vi "plot_digital.vi"(9 "array":dbl[](array[numeric]), 10 "Outputs":T1(array[cluster])=[{"Output"=0, "Offset"=0.0, "Level"=5.0, "Polarity"=TRUE, "Prescale Factor"=10, "Prescale Phase"=0, "Description"="trap open"}, {"Output"=1, "Offset"=0.0, "Level"=5.0, "Polarity"=TRUE, "Prescale Factor"=1, "Prescale Phase"=0, "Description"="scopes"}, {"Output"=2, "Offset"=0.0, "Level"=2.7, "Polarity"=TRUE, "Prescale Factor"=1, "Prescale Phase"=0, "Description"="buncher"}, {"Output"=3, "Offset"=0.0, "Level"=5.0, "Polarity"=FALSE, "Prescale Factor"=1, "Prescale Phase"=0, "Description"="q switch"}, {"Output"=4, "Offset"=0.0, "Level"=5.0, "Polarity"=TRUE, "Prescale Factor"=1, "Prescale Phase"=0, "Description"="guide"}] {"Output" items=["T0", "Output AB", "Output CD", "Output EF", "Output GH"]; "Offset" format="%#_13g"; "Prescale Phase" max=1073741822; "Prescale Factor" min=1 max=1073741823}) -> (2 "Digital Waveform Graph":digitalwaveform(graph)={"t0"=timestamp(0 s since 1904-01-01), "dt"=5.0495605468750004e-09, "Y"={"transitions"=[], "data"=array4096x5[20480 elements]}})   [LabVIEW 2015]
uses:
  <vilib>/Waveform/DWDTOps.llb/DWDT Boolean Array to Digital.vi
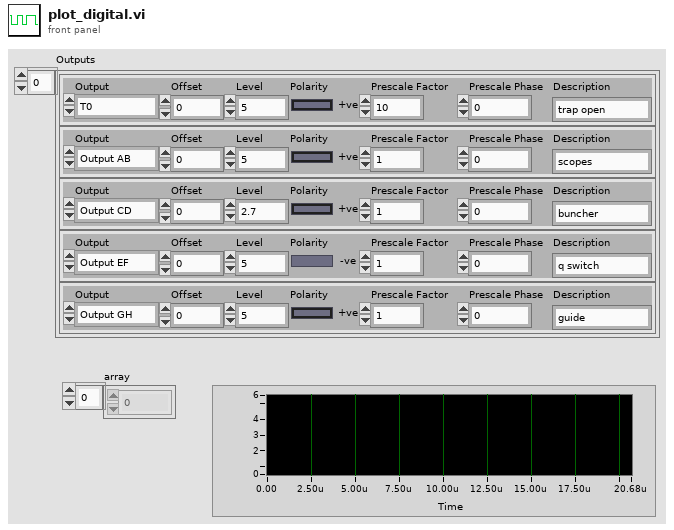
[diagram p1: front panel]
types:
  T1 = cluster{"Output":u16, "Offset":dbl, "Level":dbl, "Polarity":bool, "Prescale Factor":u32, "Prescale Phase":u32, "Description":string}[]
  T2 = cluster{"Output":u16, "Offset":dbl, "Level":dbl, "Polarity":bool, "Prescale Factor":u32, "Prescale Phase":u32, "Description":string}
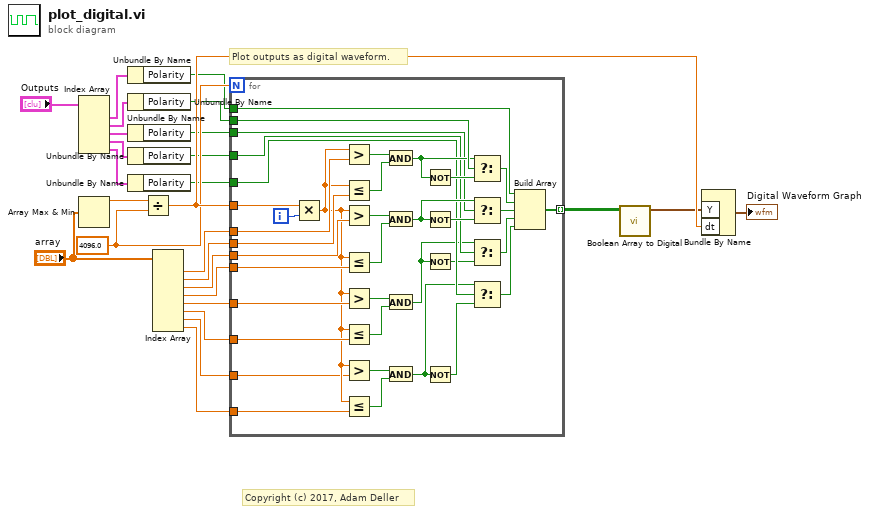
[diagram p0: block diagram]
diagram:
  w22 = 4096.0 ("y")
  # "Copyright (c) 2017, Adam Deller"
  # "Plot outputs as digital waveform."
  n1 = Index Array(array="Outputs") -> (element #1=w11:T2, element #2=w10:T2, element #3=w9:T2, element #4=w8:T2, element #5=w7:T2)  [unwired: 5 in]
  n2 = Array Max & Min(array="array") -> (max value=w23:dbl)  [unwired: 3 out]
  n3 = Unbundle By Name(w11) -> ("Polarity"=w2:bool)
  n4 = Unbundle By Name(w10) -> ("Polarity"=w3:bool)
  n5 = Unbundle By Name(w9) -> ("Polarity"=w4:bool)
  n6 = Unbundle By Name(w8) -> ("Polarity"=w5:bool)
  n7 = Unbundle By Name(w7) -> ("Polarity"=w6:bool)
  n8 = Divide(x=w23, y=w22) -> (x/y=w24:dbl)
  n9 = Index Array(array="array") -> (element #1=w21:dbl, element #2=w20:dbl, element #3=w19:dbl, element #4=w18:dbl, element #5=w17:dbl, element #6=w16:dbl, element #7=w15:dbl, element #8=w14:dbl)  [unwired: 8 in]
  n10 = for {
    N: w22 -> [_]
    tunnel: w21 -> [w59]
    tunnel: w20 -> [w58]
    tunnel: w19 -> [w55]
    tunnel: w18 -> [w54]
    tunnel: w17 -> [w51]
    tunnel: w16 -> [w50]
    tunnel: w15 -> [w45]
    tunnel: w14 -> [w46]
    tunnel: w24 -> [w60]
    tunnel: [w44] -> w13 mode=indexing
    tunnel: w3 -> [w43]
    tunnel: w4 -> [w37]
    tunnel: w5 -> [w36]
    tunnel: w6 -> [w35]
    tunnel: w2 -> [w27]
    i -> [w63]
    n11 = Multiply(x=w60, y=w63) -> (x*y=w47:dbl)
    n12 = Greater?(x=w47, y=w59) -> (0:w62:bool)
    n13 = Less Or Equal?(x=w47, y=w58) -> (x <= y?=w61:bool)
    n14 = Greater?(x=w47, y=w55) -> (0:w57:bool)
    n15 = Less Or Equal?(x=w47, y=w54) -> (x <= y?=w56:bool)
    n16 = Greater?(x=w47, y=w51) -> (0:w53:bool)
    n17 = Less Or Equal?(x=w47, y=w50) -> (x <= y?=w52:bool)
    n18 = Greater?(x=w47, y=w45) -> (0:w49:bool)
    n19 = Less Or Equal?(x=w47, y=w46) -> (x <= y?=w48:bool)
    n20 = And(x=w62, y=w61) -> (x .and. y?=w41:bool)
    n21 = And(x=w57, y=w56) -> (x .and. y?=w39:bool)
    n22 = And(x=w53, y=w52) -> (x .and. y?=w34:bool)
    n23 = And(x=w49, y=w48) -> (x .and. y?=w30:bool)
    n24 = Not(x=w41) -> (.not. x?=w40:bool)
    n25 = Not(x=w39) -> (.not. x?=w38:bool)
    n26 = Not(x=w34) -> (.not. x?=w33:bool)
    n27 = Not(x=w30) -> (.not. x?=w29:bool)
    n28 = Select(t=w41, s=w43, f=w40) -> (s? t:f=w42:bool)
    n29 = Select(t=w39, s=w37, f=w38) -> (s? t:f=w32:bool)
    n30 = Select(t=w34, s=w36, f=w33) -> (s? t:f=w31:bool)
    n31 = Select(t=w30, s=w35, f=w29) -> (s? t:f=w28:bool)
    n32 = Build Array(w27, w42, w32, w31, w28) -> (w44:bool[])
  }
  n33 = call-poly <vilib>:"Boolean Array to Digital.vi"("boolean array"=w13) -> ("digital waveform"=w12:digitalwaveform)  [unwired: 9 in, 1 out]
  n34 = Bundle By Name("Y"=w12, "dt"=w24) -> (→"Digital Waveform Graph":digitalwaveform)  [unwired: 1 in]
